vi "FG VelocityState.vi"(1 "FG Action (Read)":T3, 2 "VelocityState in":T1) -> (0 "VelocityState out":T1)   [LabVIEW 2009]
uses:
  cRIO/Functional Global Variables/Actions for FG's.ctl
  VelocityState.ctl
  TimeRec.ctl
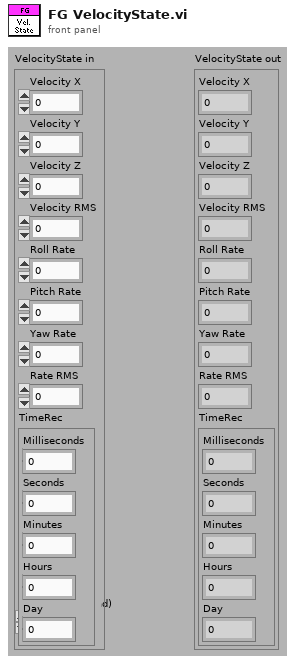
[diagram p1: front panel]
types:
  T1 = typedef "VelocityState.ctl" = cluster{"Velocity X":dbl, "Velocity Y":dbl, "Velocity Z":dbl, "Velocity RMS":dbl, "Roll Rate":dbl, "Pitch Rate":dbl, "Yaw Rate":dbl, "Rate RMS":dbl, "TimeRec":T2}
  T2 = typedef "TimeRec.ctl" = cluster{"Milliseconds":u32, "Seconds":u32, "Minutes":u32, "Hours":u32, "Day":u32}
  T3 = typedef "Actions for FG's.ctl" = enum16{"Read", "Write"}
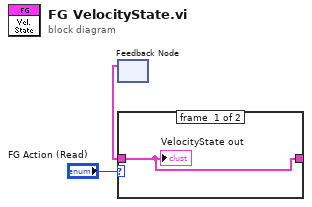
[diagram p0: block diagram]
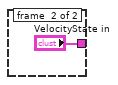
[diagram p2: hidden frame]
diagram:
  n1 = feedback #1() -> (w1:T1)  [unwired: 1 in]
  n2 = case shown="\"Write\"" "FG Action (Read)" {
    tunnel: w1 -> [w4 _]
    tunnel: [w4 "VelocityState in"] -> w2
    frame #0 {
      "VelocityState out" <- w4
    }
    frame #1 {
    }
  }
